vi "Terminated.vi"(7 "Sender":refnum<class "Sender.lvclass">, 9 "Error":errorcluster, 10 "Actor":refnum<class "Actor.lvclass">, 11 "TEMPLATE Actor in":refnum<class "TEMPLATE Actor.lvclass">) -> (0 "Error out":errorcluster, 3 "TEMPLATE Actor out":refnum<class "TEMPLATE Actor.lvclass">)   [LabVIEW 2025, in "_Template.lvlib" / "Templates.lvlib" / "TEMPLATE Actor.lvlib" / "TEMPLATE Actor.lvclass"]
uses:
  TEMPLATE Actor.lvclass
  jettl/jettl/Actor/Actor/Actor.lvclass
  jettl/jettl/Sender/Sender/Sender.lvclass
  TEMPLATE Actor.lvclass/TEMPLATE Actor.ctl
  jettl/jettl/Terminated Msg/Terminated Msg.lvlib
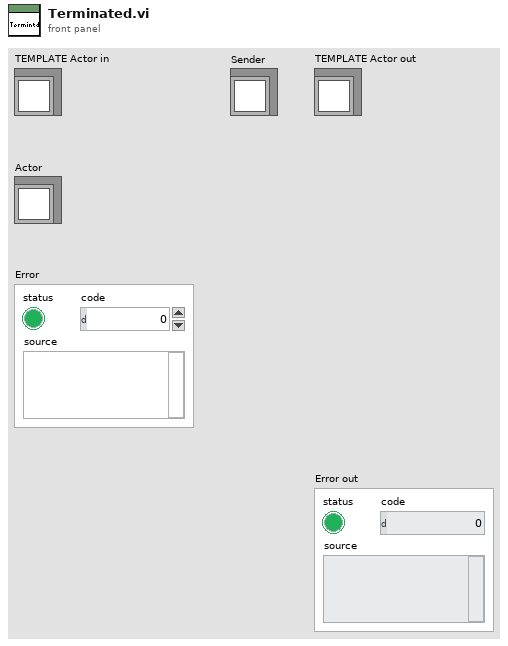
[diagram p1: front panel]
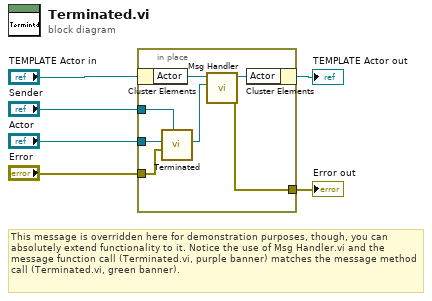
[diagram p0: block diagram]
diagram:
  # "This message is overridden here for demonstration purposes, though, you can absolutely extend functionality to it. Notice the use of Msg Handler.vi and the message function call (Terminated.vi, purple banner) matches the message method call (Terminated.vi, green banner)."
  n1 = in-place {
    in-place-border: [w11] -> w4
    in-place-border: "Sender" -> [w10]
    in-place-border: "Error" -> [w9]
    in-place-border: "Actor" -> [w8]
    n2 = in-place-cluster #1("TEMPLATE Actor in") -> ("Actor"=w13:refnum<class "Actor.lvclass">)
    n3 = call "Terminated.vi"("Sender"=w10, "Error"=w9, "Actor"=w8) -> ("Msg"=w7:refnum<class "Msg.lvclass">)  [unwired: 8 in]
    n4 = call-dynamic "Msg Handler.vi"("Msg"=w7, "Actor in"=w13) -> ("Error out"=w11:errorcluster, "Actor out"=w12:refnum<class "Actor.lvclass">)  [unwired: 8 in]
    n5 = in-place-cluster #1("Actor"=w12) -> (→"TEMPLATE Actor out":refnum<class "TEMPLATE Actor.lvclass">)
  }
  "Error out" <- w4
